vi "json test.vi"() -> ()   [LabVIEW 2016]
uses:
  Dashboard Control.ctl
panel:
  out "JSON string":string
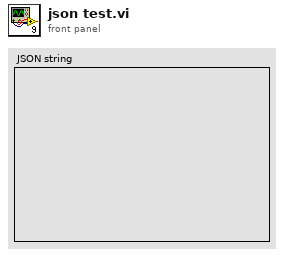
[diagram p1: front panel]
types:
  T1 = typedef "Dashboard Control.ctl" = cluster{"Tractive System":bool, "RTD":bool, "AMS error":bool, "IMD error":bool, "Low Voltage":dbl, "High Voltage":dbl}
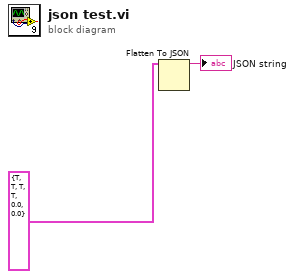
[diagram p0: block diagram]
diagram:
  n1 = Flatten To JSON(anything=T1 {"Tractive System"=TRUE, "RTD"=TRUE, "AMS error"=TRUE, "IMD error"=TRUE, "Low Voltage"=0.0, "High Voltage"=0.0} ("Dashboard Control")) -> (JSON string=→"JSON string":string)  [unwired: 2 in, 1 out]
